vi "Acquire PWM.vi"(9 "Connector m Bank n Settings":T4={"PWM 0 Settings"={"ACTIVE EDGE"=TRUE, "TIMEOUT"=40000000}, "PWM 1 Settings"={"ACTIVE EDGE"=TRUE, "TIMEOUT"=40000000}, "PWM 2 Settings"={"ACTIVE EDGE"=TRUE, "TIMEOUT"=40000000}, "PWM 3 Settings"={"ACTIVE EDGE"=TRUE, "TIMEOUT"=40000000}, "PWM 4 Settings"={"ACTIVE EDGE"=TRUE, "TIMEOUT"=40000000}, "PWM 5 Settings"={"ACTIVE EDGE"=TRUE, "TIMEOUT"=40000000}, "PWM 6 Settings"={"ACTIVE EDGE"=TRUE, "TIMEOUT"=40000000}, "PWM 7 Settings"={"ACTIVE EDGE"=TRUE, "TIMEOUT"=40000000}}, 11 "Bank in":refnum<class "Bank.lvclass">) -> (1 "Connector m Bank n PWM Acquisition":T1, 3 "Bank out":refnum<class "Bank.lvclass">)   [LabVIEW 2019, in "LRUTS FPGA IP.lvlib" / "Bank.lvclass"]
uses:
  Bank.lvclass
  PWM Acquisition Bank Settings.ctl
  PWM Acquisition Channel Settings.ctl
  PWM Acquisition Bank Results.ctl
  PWM Acquisition Channel Results.ctl
  PWM Acquisition Channel Measurement.ctl
  Bank Type.ctl
  Bank.lvclass/Bank.ctl
  <vilib>/rvi/eio/common/nirviEmuTemplateMethod_errors.vi
  <vilib>/eio/EIONode/EIONode.xnode
  <instrlib>/_niInstr/Basic Elements/v1/FPGA/niInstr Basic Elements v1 FPGA.lvlib
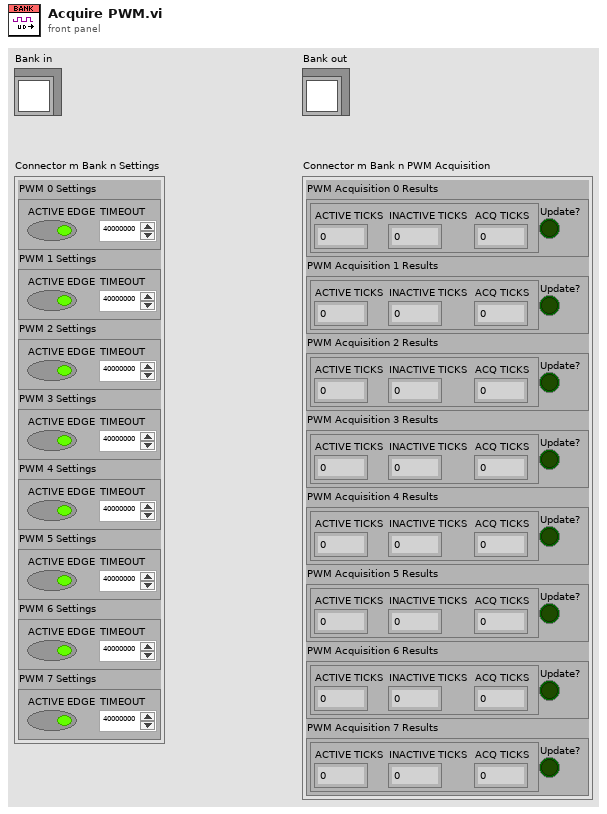
[diagram p1: front panel]
types:
  T1 = typedef "LRUTS FPGA IP.lvlib/Bank.lvclass/PWM Acquisition Bank Results.ctl" = cluster{"PWM Acquisition 0 Results":T2, "PWM Acquisition 1 Results":T2, "PWM Acquisition 2 Results":T2, "PWM Acquisition 3 Results":T2, "PWM Acquisition 4 Results":T2, "PWM Acquisition 5 Results":T2, "PWM Acquisition 6 Results":T2, "PWM Acquisition 7 Results":T2}
  T2 = typedef "LRUTS FPGA IP.lvlib/Bank.lvclass/PWM Acquisition Channel Results.ctl" = cluster{"Measurement":T3, "Update?":bool}
  T3 = typedef "LRUTS FPGA IP.lvlib/Bank.lvclass/PWM Acquisition Channel Measurement.ctl" = cluster{"ACTIVE TICKS":u32, "INACTIVE TICKS":u32, "ACQ TICKS":u32}
  T4 = typedef "LRUTS FPGA IP.lvlib/Bank.lvclass/PWM Acquisition Bank Settings.ctl" = cluster{"PWM 0 Settings":T5, "PWM 1 Settings":T5, "PWM 2 Settings":T5, "PWM 3 Settings":T5, "PWM 4 Settings":T5, "PWM 5 Settings":T5, "PWM 6 Settings":T5, "PWM 7 Settings":T5}
  T5 = typedef "LRUTS FPGA IP.lvlib/Bank.lvclass/PWM Acquisition Channel Settings.ctl" = cluster{"ACTIVE EDGE":bool, "TIMEOUT":u32}
  T6 = typedef "LRUTS FPGA IP.lvlib/Bank.lvclass/Bank Type.ctl" = enum16{"None", "Discrete Acquisition", "Discrete Generation", "PWM Acquisition", "PWM Generation"}
  T7 = typedef "LRUTS FPGA IP.lvlib/Bank.lvclass/FPGA IO Resources.ctl" = cluster{"DIO 0":refnum<k21>, "DIO 1":refnum<k21>, "DIO 2":refnum<k21>, "DIO 3":refnum<k21>, "DIO 4":refnum<k21>, "DIO 5":refnum<k21>, "DIO 6":refnum<k21>, "DIO 7":refnum<k21>}
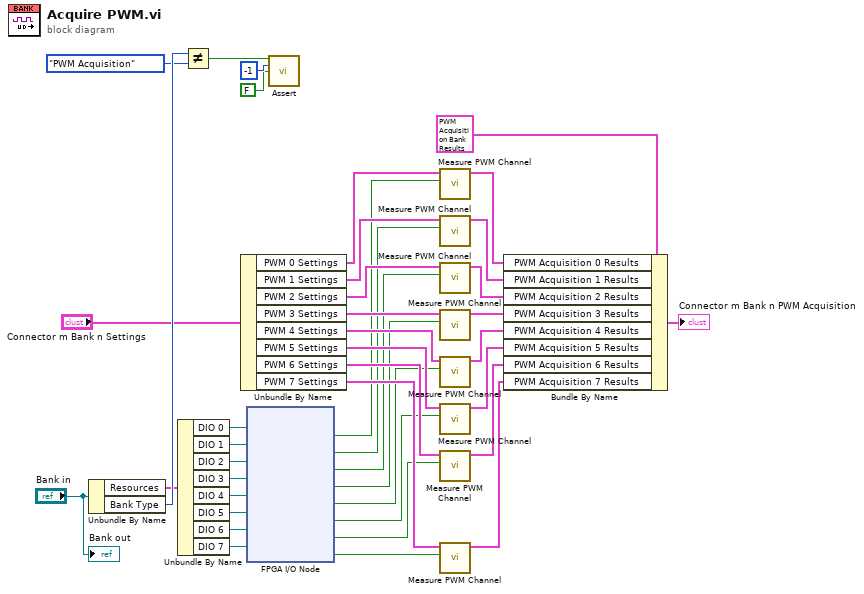
[diagram p0: block diagram]
diagram:
  n1 = Unbundle By Name("Bank in") -> ("Resources"=w36:T7, "Bank Type"=w41:T6)
  n2 = Unbundle By Name(w36) -> ("DIO 0"=w35:refnum<k21>, "DIO 1"=w34:refnum<k21>, "DIO 2"=w33:refnum<k21>, "DIO 3"=w32:refnum<k21>, "DIO 4"=w31:refnum<k21>, "DIO 5"=w30:refnum<k21>, "DIO 6"=w29:refnum<k21>, "DIO 7"=w28:refnum<k21>)
  n3 = Not Equal?(x=w41, y=Bank_Type."PWM Acquisition") -> (x != y?=w39:bool)
  n4 = Unbundle By Name("Connector m Bank n Settings") -> ("PWM 0 Settings"=w26:T5, "PWM 1 Settings"=w25:T5, "PWM 2 Settings"=w24:T5, "PWM 3 Settings"=w23:T5, "PWM 4 Settings"=w22:T5, "PWM 5 Settings"=w21:T5, "PWM 6 Settings"=w20:T5, "PWM 7 Settings"=w19:T5)
  n5 = xnode "FPGA I/O Node"("FPGA I/O In"=w35, "FPGA I/O In"=w34, "FPGA I/O In"=w33, "FPGA I/O In"=w32, "FPGA I/O In"=w31, "FPGA I/O In"=w30, "FPGA I/O In"=w29, "FPGA I/O In"=w28) -> ("I/O Item"=w18:bool, "I/O Item"=w17:bool, "I/O Item"=w16:bool, "I/O Item"=w15:bool, "I/O Item"=w14:bool, "I/O Item"=w13:bool, "I/O Item"=w12:bool, "I/O Item"=w11:bool)  [unwired: 8 out]
  n6 = call <instrlib>:"Assert.vi"("assert"=w39, "error code"=-1, "enable show error"=FALSE) -> ()  [unwired: 13 in]
  n7 = call "Measure PWM Channel.vi"("State"=w18, "Settings"=w26) -> ("Results"=w9:T2)  [unwired: 9 in]
  n8 = call "Measure PWM Channel.vi"("State"=w17, "Settings"=w25) -> ("Results"=w8:T2)  [unwired: 9 in]
  n9 = call "Measure PWM Channel.vi"("State"=w16, "Settings"=w24) -> ("Results"=w7:T2)  [unwired: 9 in]
  n10 = call "Measure PWM Channel.vi"("State"=w15, "Settings"=w23) -> ("Results"=w6:T2)  [unwired: 9 in]
  n11 = call "Measure PWM Channel.vi"("State"=w14, "Settings"=w22) -> ("Results"=w5:T2)  [unwired: 9 in]
  n12 = call "Measure PWM Channel.vi"("State"=w13, "Settings"=w21) -> ("Results"=w4:T2)  [unwired: 9 in]
  n13 = call "Measure PWM Channel.vi"("State"=w12, "Settings"=w20) -> ("Results"=w3:T2)  [unwired: 9 in]
  n14 = call "Measure PWM Channel.vi"("State"=w11, "Settings"=w19) -> ("Results"=w2:T2)  [unwired: 9 in]
  n15 = Bundle By Name(cluster=T1 {"PWM Acquisition 0 Results"={"Measurement"={"ACTIVE TICKS"=0, "INACTIVE TICKS"=0, "ACQ TICKS"=0}, "Update?"=FALSE}, "PWM Acquisition 1 Results"={"Measurement"={"ACTIVE TICKS"=0, "INACTIVE TICKS"=0, "ACQ TICKS"=0}, "Update?"=FALSE}, "PWM Acquisition 2 Results"={"Measurement"={"ACTIVE TICKS"=0, "INACTIVE TICKS"=0, "ACQ TICKS"=0}, "Update?"=FALSE}, "PWM Acquisition 3 Results"={"Measurement"={"ACTIVE TICKS"=0, "INACTIVE TICKS"=0, "ACQ TICKS"=0}, "Update?"=FALSE}, "PWM Acquisition 4 Results"={"Measurement"={"ACTIVE TICKS"=0, "INACTIVE TICKS"=0, "ACQ TICKS"=0}, "Update?"=FALSE}, "PWM Acquisition 5 Results"={"Measurement"={"ACTIVE TICKS"=0, "INACTIVE TICKS"=0, "ACQ TICKS"=0}, "Update?"=FALSE}, "PWM Acquisition 6 Results"={"Measurement"={"ACTIVE TICKS"=0, "INACTIVE TICKS"=0, "ACQ TICKS"=0}, "Update?"=FALSE}, "PWM Acquisition 7 Results"={"Measurement"={"ACTIVE TICKS"=0, "INACTIVE TICKS"=0, "ACQ TICKS"=0}, "Update?"=FALSE}} ("PWM Acquisition Bank Results"), "PWM Acquisition 0 Results"=w9, "PWM Acquisition 1 Results"=w8, "PWM Acquisition 2 Results"=w7, "PWM Acquisition 3 Results"=w6, "PWM Acquisition 4 Results"=w5, "PWM Acquisition 5 Results"=w4, "PWM Acquisition 6 Results"=w3, "PWM Acquisition 7 Results"=w2) -> (→"Connector m Bank n PWM Acquisition":T1)
  "Bank out" <- "Bank in"
